vi "GPS Read VISA Instance.vi"(0 "VISA In":refnum<visa-resource-name>, 1 "Buffer In":string, 5 "Error In":errorcluster) -> (13 "Output Valid?":bool, 14 "VISA Out":refnum<visa-resource-name>, 15 "Buffer Out":string, 16 "Time":dbl, 17 "Longitude":dbl, 18 "Latitude":dbl, 19 "Error Out":errorcluster)   [LabVIEW 2009]
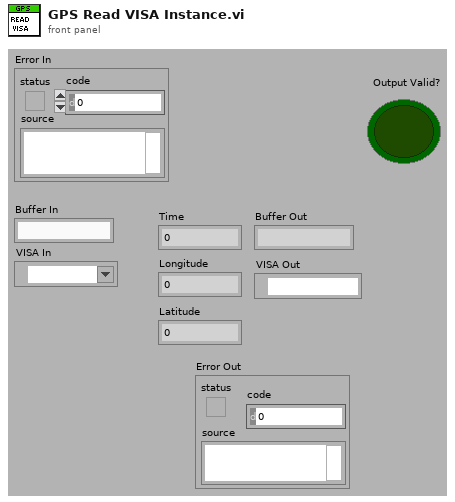
[diagram p1: front panel]
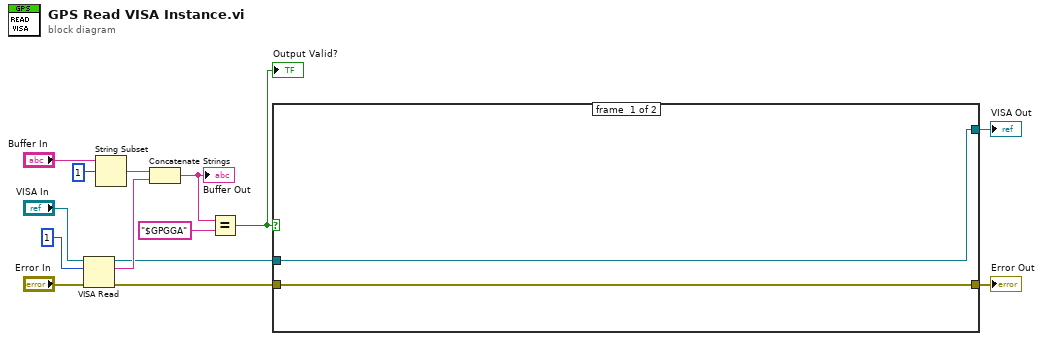
[diagram p0: block diagram]
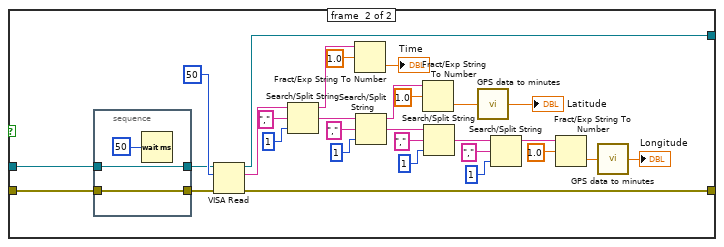
[diagram p2: hidden frame]
diagram:
  n1 = VISA Read(VISA resource name="VISA In", byte count=u32 1, error in (no error)="Error In") -> (VISA resource name out=w6:refnum<visa-resource-name>, read buffer=w12:string, error out=w7:errorcluster)  [unwired: 1 out]
  n2 = String Subset(string="Buffer In", offset (0)=1) -> (substring=w11:string)  [unwired: 1 in]
  n3 = Concatenate Strings(w11, w12) -> (w10:string)
  "Buffer Out" <- w10
  n4 = Equal?(x=w10, y="$GPGGA") -> (x = y?=w8:bool)
  "Output Valid?" <- w8
  n5 = case shown="True" w8 {
    tunnel: w6 -> [w16 w18]
    tunnel: w7 -> [w15 w20]
    tunnel: [w16 w34] -> w1
    tunnel: [w15 w33] -> w2
    frame #0 {
    }
    frame #1 {
      n6 = stacked-sequence {
        tunnel: w20 -> [w49]
        tunnel: [w49] -> w19
        tunnel: w18 -> [w48]
        tunnel: [w48] -> w17
        frame #0 {
          n7 = Wait (ms)(milliseconds to wait=u32 50) -> ()  [unwired: 1 out]
        }
      }
      n8 = VISA Read(VISA resource name=w17, byte count=u32 50, error in (no error)=w19) -> (VISA resource name out=w34:refnum<visa-resource-name>, read buffer=w32:string, error out=w33:errorcluster)  [unwired: 1 out]
      n9 = Search/Split String(string=w32, search string/char (-)=",", offset (0)=1) -> (substring before match=w28:string, match + rest of string=w39:string)  [unwired: 1 out]
      n10 = Fract/Exp String To Number(string=w28, offset=1.0 ("default (0 I32)")) -> (number=→"Time":dbl)  [unwired: 2 in, 1 out]
      n11 = Search/Split String(string=w39, search string/char (-)=",", offset (0)=1) -> (substring before match=w31:string, match + rest of string=w38:string)  [unwired: 1 out]
      n12 = Fract/Exp String To Number(string=w31, offset=1.0 ("default (0 DBL)")) -> (number=w24:dbl)  [unwired: 2 in, 1 out]
      n13 = Search/Split String(string=w38, search string/char (-)=",", offset (0)=1) -> (match + rest of string=w35:string)  [unwired: 2 out]
      n14 = call "GPS data to minutes.vi"("GPS Data in (DDmm.mm)"=w24) -> ("GPS Data out (in minutes)"=→"Latitude":dbl)
      n15 = Search/Split String(string=w35, search string/char (-)=",", offset (0)=1) -> (substring before match=w29:string)  [unwired: 2 out]
      n16 = Fract/Exp String To Number(string=w29, offset=1.0 ("default (0 I32)")) -> (number=w22:dbl)  [unwired: 2 in, 1 out]
      n17 = call "GPS data to minutes.vi"("GPS Data in (DDmm.mm)"=w22) -> ("GPS Data out (in minutes)"=→"Longitude":dbl)
    }
  }
  "Error Out" <- w2
  "VISA Out" <- w1
